vi "Determine Warnings.viexercise 3-8.vi"() -> ()   [LabVIEW 2014]
panel:
  out "Warning?":bool
  out "Warning Text":string
  in  "Current Temp":dbl
  in  "Max Temp":dbl
  in  "Min Temp":dbl
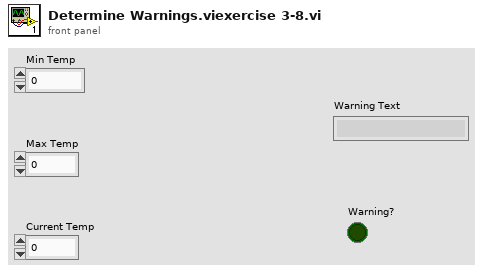
[diagram p1: front panel]
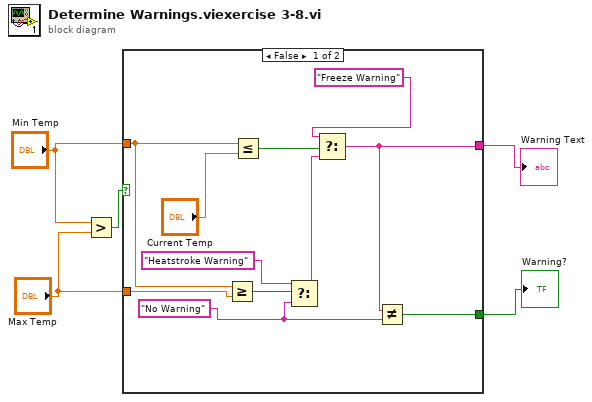
[diagram p0: block diagram]
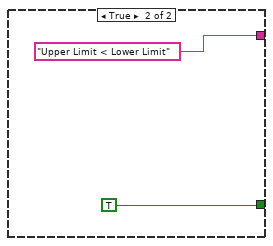
[diagram p2: hidden frame]
diagram:
  n1 = Greater?(x="Min Temp", y="Max Temp") -> (0:w2:bool)
  n2 = case shown="False" w2 {
    tunnel: "Min Temp" -> [w8 _]
    tunnel: [w13 TRUE] -> w4
    tunnel: [w9 "Upper Limit < Lower Limit"] -> w3
    tunnel: "Max Temp" -> [w7 _]
    frame False {
      w15 = "No Warning"
      n3 = Greater Or Equal?(x=w8, y=w7) -> (x >= y?=w6:bool)
      n4 = Less Or Equal?(x=w8, y="Current Temp") -> (x <= y?=w10:bool)
      n5 = Select(t="Heatstroke Warning", s=w6, f=w15) -> (s? t:f=w11:string)
      n6 = Select(t="Freeze Warning", s=w10, f=w11) -> (s? t:f=w9:string)
      n7 = Not Equal?(x=w9, y=w15) -> (x != y?=w13:bool)
    }
    frame True {
    }
  }
  "Warning Text" <- w3
  "Warning?" <- w4
